vi "VariablesToString.vi"   [LabVIEW 2011]
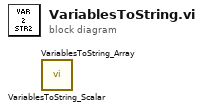
[diagram p0: block diagram]
diagram:
  n1 = call "VariablesToString_Scalar.vi"() -> ()  [unwired: 3 in, 1 out]
  n2 = call "VariablesToString_Array.vi"() -> ()  [unwired: 3 in, 1 out]
